vi "TLPM VXIpnp Error Converter.vi"(8 "error in (no error)":errorcluster {"code" format="%.0x"}, 9 "Name Of VI (\"\")":string, 10 "CVI Error Code (0)":i32 format="%.0x", 11 "instrument handle":u32) -> (0 "error out":errorcluster {"code" format="%.0x"}, 3 "instrument handle out":u32)   [LabVIEW 2019]
doc: "This VI converts error codes from VXIPnp instrument driver to standard LabVIEW error codes. If an error is detected the VI builds the appropriate error cluster that is readable by one of the error handlers supplied with LabVIEW."
uses:
  TLPM_32.dll
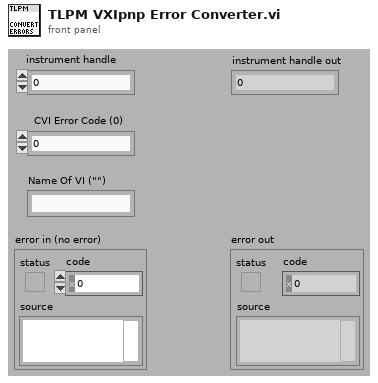
[diagram p1: front panel]
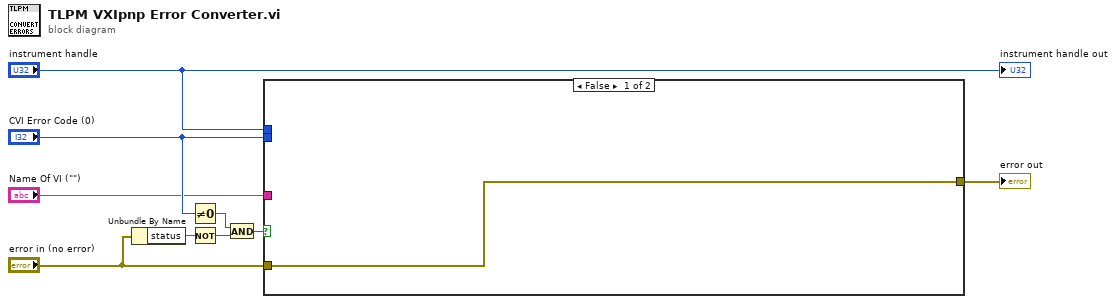
[diagram p0: block diagram]
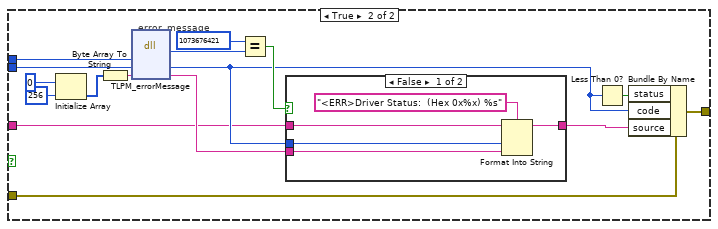
[diagram p2: hidden frame]
diagram:
  n1 = Unbundle By Name("error in (no error)") -> ("status"=w8:bool)
  n2 = Not Equal To 0?(x="CVI Error Code (0)") -> (x != 0?=w9:bool)
  n3 = Not(x=w8) -> (.not. x?=w6:bool)
  n4 = And(x=w9, y=w6) -> (x .and. y?=w7:bool)
  n5 = case shown="False" w7 {
    tunnel: "CVI Error Code (0)" -> [_ w26]
    tunnel: [w10 w25] -> w4
    tunnel: "error in (no error)" -> [w10 w24]
    tunnel: "instrument handle" -> [_ w19]
    tunnel: "Name Of VI (\"\")" -> [_ w11]
    frame False {
    }
    frame True {
      # "error_message"
      n6 = Initialize Array(u8 0, 256) -> (w22:u8[])
      n7 = Byte Array To String(unsigned byte array=w22) -> (string=w20:string)
      n8 = dll-call lib="TLPM_32.dll" fn="TLPM_errorMessage"(w19, w26, w20) -> (w17:i32, w12:i32, w15:string)  [unwired: 4 in, 2 out]
      n9 = Equal?(x=1073676421 ("y"), y=w17) -> (x = y?=w16:bool)
      n10 = case shown="False" w16 {
        tunnel: w15 -> [w29 _]
        tunnel: w11 -> [w31 w32]
        tunnel: w12 -> [w30 _]
        tunnel: [w28 w32] -> w14
        frame False {
          n11 = Format Into String(format string="<ERR>Driver Status:  (Hex 0x%x) %s", initial string=w31, w30, w29) -> (resulting string=w28:string)  [unwired: 1 in, 1 out]
        }
        frame True {
        }
      }
      n12 = Less Than 0?(x=w12) -> (x < 0?=w13:bool)
      n13 = Bundle By Name(cluster=w24, "status"=w13, "code"=w12, "source"=w14) -> (w25:errorcluster)
    }
  }
  "error out" <- w4
  "instrument handle out" <- "instrument handle"
